vi "ContourPlot v3.5-dist.vi"() -> ()   [LabVIEW 2018]
uses:
  <vilib>/Utility/file.llb/Read Delimited Spreadsheet (DBL).vi
  <vilib>/Analysis/NI_AALBase.lvlib
panel:
  in  "Specify file name":string
  out "Ready?":bool=TRUE
  in  "Tab Control 2":enum32{"Contour"}(tab)
  out "Intensity Graph":dbl[][](graph)
  in  "Tab Control":enum32{"IV", "Y curve"}(tab)=enum."Y curve"
  out "IV":cluster{dbl[], "Intensity Graph":dbl[]}(graph)
  in  "intervals":i32=100
  out "Y Histogram":T1(graph)={"X Values"=[1.37164696, 1.37617088, 1.3806948, 1.3852187200000001, 1.3897426400000001, 1.3942665600000002, 1.3987904800000002, 1.4033144000000002, 1.4078383200000002, 1.4123622400000002, 1.4168861600000002, 1.4214100800000002, 1.4259340000000003, 1.4304579200000003, 1.4349818400000003, 1.4395057600000003, 1.4440296800000003, 1.4485536000000003, 1.4530775200000003, 1.4576014400000004, 1.4621253600000004, 1.4666492800000004, 1.4711732000000004, 1.4756971200000004, 1.4802210400000004, 1.4847449600000004, 1.4892688800000005, 1.4937928000000005, 1.4983167200000005, 1.5028406400000005, 1.5073645600000005, 1.5118884800000005, 1.5164124000000005, 1.5209363200000006, 1.5254602400000006, 1.5299841600000006, 1.5345080800000006, 1.5390320000000006, 1.5435559200000006, 1.5480798400000007, 1.5526037600000007, 1.5571276800000007, 1.5616516000000007, 1.5661755200000007, 1.5706994400000007, 1.5752233600000007, 1.5797472800000008, 1.5842712000000008, 1.5887951200000008, 1.5933190400000008, 1.5978429600000008, 1.6023668800000008, 1.6068908000000008, 1.6114147200000009, 1.6159386400000009, 1.6204625600000009, 1.624986480000001, 1.629510400000001, 1.634034320000001, 1.638558240000001, 1.643082160000001, 1.647606080000001, 1.652130000000001, 1.656653920000001, 1.661177840000001, 1.665701760000001, 1.670225680000001, 1.674749600000001, 1.679273520000001, 1.683797440000001, 1.688321360000001, 1.6928452800000011, 1.6973692000000011, 1.7018931200000011, 1.7064170400000012, 1.7109409600000012, 1.7154648800000012, 1.7199888000000012, 1.7245127200000012, 1.7290366400000012, 1.7335605600000012, 1.7380844800000013, 1.7426084000000013, 1.7471323200000013, 1.7516562400000013, 1.7561801600000013, 1.7607040800000013, 1.7652280000000014, 1.7697519200000014, 1.7742758400000014, 1.7787997600000014, 1.7833236800000014, 1.7878476000000014, 1.7923715200000014, 1.7968954400000015, 1.8014193600000015, 1.8059432800000015, 1.8104672000000015, 1.8149911200000015, 1.8195150400000015], "Histogram: h(x)"=[1, 0, 0, 0, 0, 0, 0, 0, 0, 0, 0, 0, 0, 1, 1, 0, 2, 2, 2, 4, 0, 3, 6, 3, 1, 3, 6, 4, 6, 15, 8, 11, 6, 9, 13, 14, 15, 20, 14, 33, 26, 25, 43, 24, 68, 59, 47, 54, 80, 55, 97, 117, 84, 123, 108, 186, 155, 136, 172, 226, 149, 210, 256, 185, 203, 197, 296, 250, 161, 231, 242, 182, 279, 287, 175, 211, 190, 344, 289, 192, 282, 347, 242, 329, 390, 235, 260, 214, 299, 206, 137, 141, 129, 50, 53, 27, 20, 11, 4, 7]}
  in  "Histogram range":dbl=0.4
  in  "book number":i32=416
  in  "file path (dialog if empty)":path=path "C:/Users/gyue/Box Sync/Guang Yue/data/Contour plot"
  # "Default: Empty"
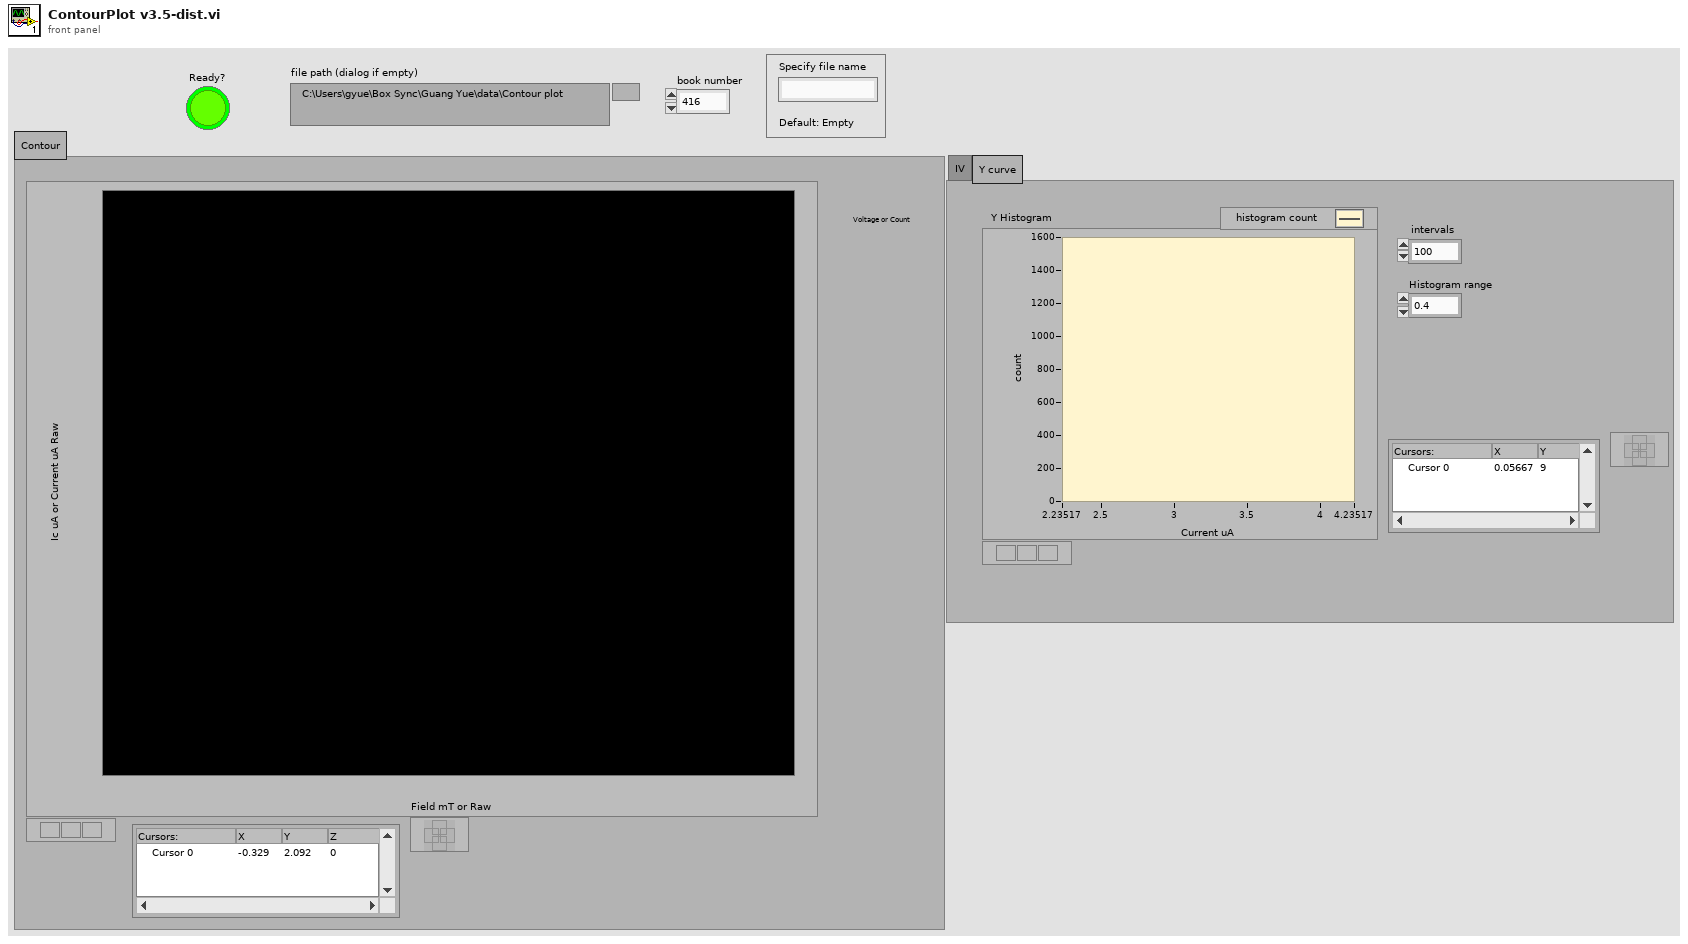
[diagram p1: front panel]
types:
  T1 = cluster{"X Values":dbl[], "Histogram: h(x)":i32[]}
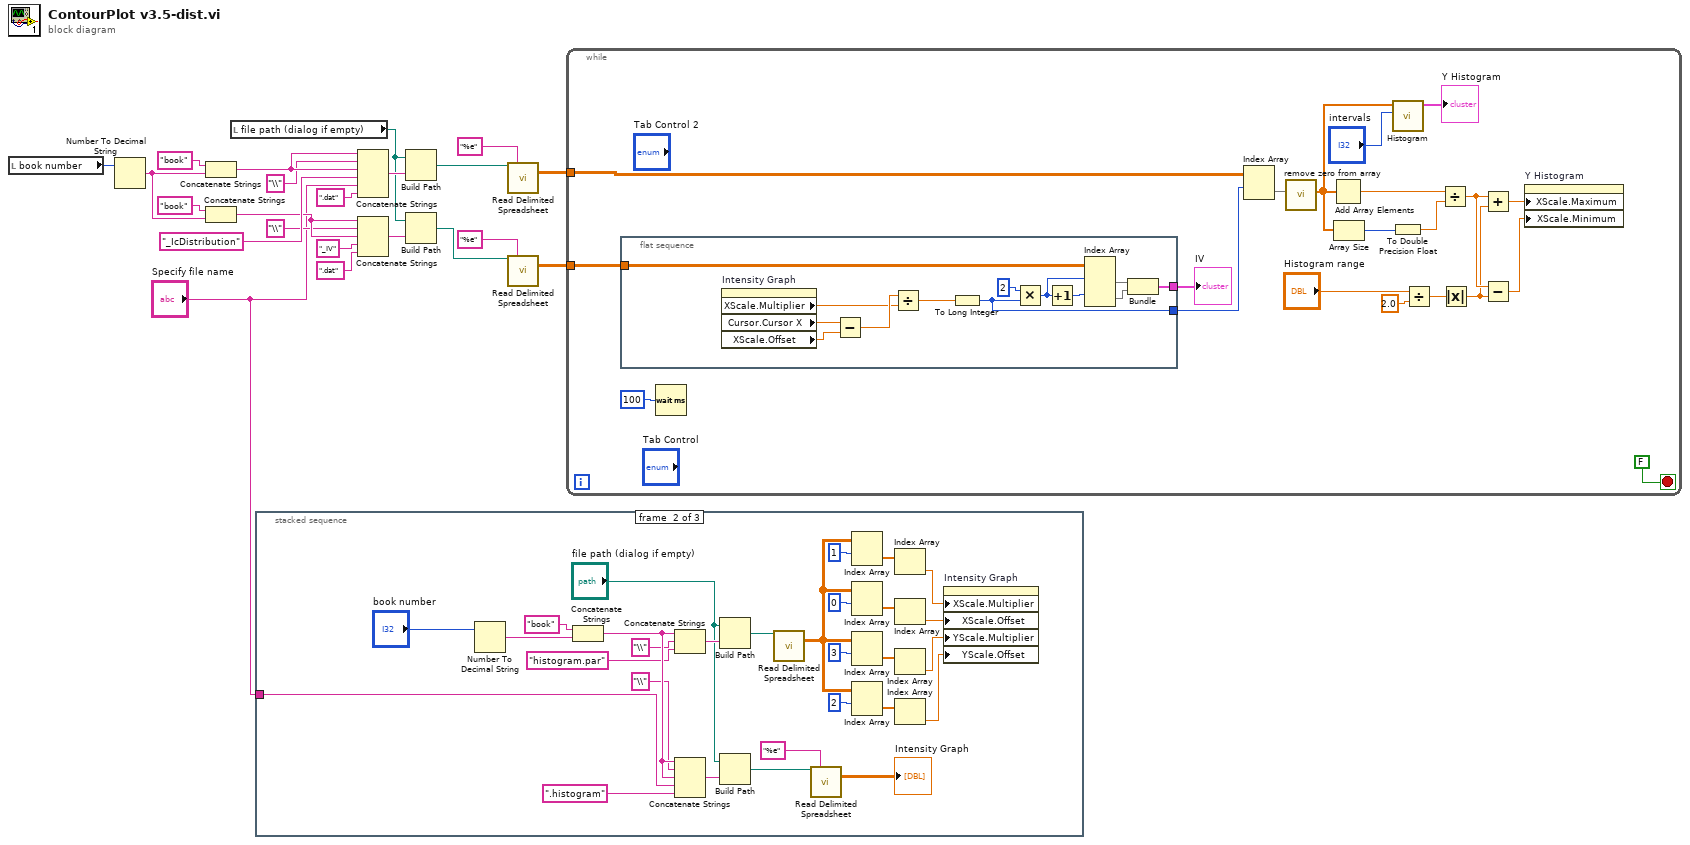
[diagram p0: block diagram]
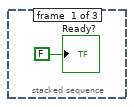
[diagram p2: hidden frame]
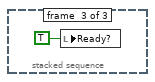
[diagram p3: hidden frame]
diagram:
  n1 = local read "book number"() -> (w18:i32)
  n2 = Number To Decimal String(number=w18) -> (decimal integer string=w5:string)  [unwired: 1 in]
  n3 = Concatenate Strings("book" ("string"), w5) -> (w19:string)
  n4 = Concatenate Strings("book" ("string"), w5) -> (w11:string)
  n5 = local read "file path (dialog if empty)"() -> (w3:path)
  n6 = stacked-sequence {
    tunnel: "Specify file name" -> [_ w24 _]
    frame #0 {
      "Ready?" <- FALSE ("Ready?")
    }
    frame #1 {
      n7 = Number To Decimal String(number="book number") -> (decimal integer string=w48:string)  [unwired: 1 in]
      n8 = Concatenate Strings("book" ("string"), w48) -> (w30:string)
      n9 = Concatenate Strings(w30, "\\" ("string"), "histogram.par" ("string")) -> (w50:string)
      n10 = Concatenate Strings(w30, "\\" ("string"), w30, w24, ".histogram" ("string")) -> (w49:string)
      n11 = Build Path(base path="file path (dialog if empty)", name or relative path=w50) -> (appended path=w51:path)
      n12 = Build Path(base path="file path (dialog if empty)", name or relative path=w49) -> (appended path=w52:path)
      n13 = call-poly <vilib>:"Read Delimited Spreadsheet.vi"("file path (dialog if empty)"=w51) -> ("all rows"=w44:dbl[][])  [unwired: 9 in, 5 out]
      n14 = call-poly <vilib>:"Read Delimited Spreadsheet.vi"("file path (dialog if empty)"=w52, "format (%.3f)"="%e") -> ("all rows"=→"Intensity Graph":dbl[][])  [unwired: 8 in, 5 out]
      n15 = Index Array(array=w44, index (row)=1) -> (element=w40:dbl[])  [unwired: 1 in]
      n16 = Index Array(array=w44, index (row)=0) -> (element=w41:dbl[])  [unwired: 1 in]
      n17 = Index Array(array=w44, index (row)=3) -> (element=w38:dbl[])  [unwired: 1 in]
      n18 = Index Array(array=w44, index (row)=2) -> (element=w39:dbl[])  [unwired: 1 in]
      n19 = Index Array(array=w40) -> (element=w31:dbl)  [unwired: 1 in]
      n20 = Index Array(array=w41) -> (element=w32:dbl)  [unwired: 1 in]
      n21 = Index Array(array=w38) -> (element=w33:dbl)  [unwired: 1 in]
      n22 = Index Array(array=w39) -> (element=w34:dbl)  [unwired: 1 in]
      n23 = property on="Intensity Graph" class="IntGraph (strict)"("XScale.Multiplier"=w31, "XScale.Offset"=w32, "YScale.Multiplier"=w33, "YScale.Offset"=w34) -> ()  [unwired: 2 in, 2 out]
    }
    frame #2 {
      n24 = local write "Ready?"(TRUE ("Ready?")) -> ()
    }
  }
  n25 = Concatenate Strings(w19, "\\" ("string"), w19, "_IcDistribution" ("string"), "Specify file name", ".dat" ("string")) -> (w20:string)
  n26 = Concatenate Strings(w11, "\\" ("string"), w11, "_IV" ("string"), ".dat" ("string")) -> (w12:string)
  n27 = Build Path(base path=w3, name or relative path=w20) -> (appended path=w21:path)
  n28 = Build Path(base path=w3, name or relative path=w12) -> (appended path=w13:path)
  n29 = call-poly <vilib>:"Read Delimited Spreadsheet.vi"("file path (dialog if empty)"=w21, "format (%.3f)"="%e") -> ("all rows"=w22:dbl[][])  [unwired: 8 in, 5 out]
  n30 = call-poly <vilib>:"Read Delimited Spreadsheet.vi"("file path (dialog if empty)"=w13, "format (%.3f)"="%e") -> ("all rows"=w4:dbl[][])  [unwired: 8 in, 5 out]
  n31 = while {
    tunnel: w22 -> [w69]
    tunnel: w4 -> [w66]
    stop <- FALSE stop-if-true
    n32 = flat-sequence {
      tunnel: [w82] -> w73
      tunnel: [w74] -> w70
      tunnel: w66 -> [w79]
      frame #0 {
        n33 = property on="Intensity Graph" class="IntGraph (strict)"() -> ("XScale.Multiplier"=w85:dbl, "Cursor.Cursor X"=w84:dbl, "XScale.Offset"=w83:dbl)  [unwired: 2 in, 2 out]
        n34 = Subtract(x=w84, y=w83) -> (x-y=w86:dbl)
        n35 = Divide(x=w86, y=w85) -> (x/y=w81:dbl)
        n36 = To Long Integer(number=w81) -> (32bit integer=w74:i32)
        n37 = Multiply(x=2, y=w74) -> (x*y=w77:i32)
        n38 = Increment(x=w77) -> (x+1=w76:i32)
        n39 = Index Array(array=w79, index (row) #1=w77, index (row) #2=w76) -> (element #1=w78:dbl[], element #2=w75:dbl[])  [unwired: 2 in]
        n40 = Bundle("all rows"=w78, "all rows"=w75) -> (w82:cluster{"all rows":dbl[], "all rows":dbl[]})  [unwired: 1 in]
      }
    }
    n41 = Wait (ms)(milliseconds to wait=u32 100) -> ()  [unwired: 1 out]
    n42 = Index Array(array=w69, index (row)=w70) -> (element=w55:dbl[])  [unwired: 1 in]
    n43 = call "remove zero from array.vi"("in"=w55) -> ("out"=w54:dbl[])  [unwired: 10 in]
    n44 = Add Array Elements(numeric array=w54) -> (sum=w63:dbl)
    n45 = Array Size(array=w54) -> (size(s)=w62:i32)
    n46 = call <vilib>:"Histogram.vi"("intervals"="intervals", "X"=w54) -> ("Histogram Graph"=→"Y Histogram":T1)  [unwired: 6 in, 3 out]
    n47 = To Double Precision Float(number=w62) -> (double precision float=w61:dbl)
    n48 = Divide(x="Histogram range", y=2.0) -> (x/y=w60:dbl)
    n49 = Divide(x=w63, y=w61) -> (x/y=w58:dbl)
    n50 = Absolute Value(x=w60) -> (abs(x)=w57:dbl)
    n51 = Add(x=w58, y=w57) -> (x+y=w59:dbl)
    n52 = Subtract(x=w58, y=w57) -> (x-y=w56:dbl)
    n53 = property on="Y Histogram" class="XYGraph (strict)"("XScale.Maximum"=w59, "XScale.Minimum"=w56) -> ()  [unwired: 2 in, 2 out]
    "IV" <- w73
  }
